vi "LVClass_SlopesPostProcessList ctor from copy.vi"(0 "SlopesPostProcessorList (const)":refnum<class "SlopesPostProcessorList.lvclass">, 5 "Dimensions_um":T1={"Size"={"X"=32, "Y"=32}, "Step"={"X"=1.0, "Y"=1.0}}, 7 "serial":string="7102", 9 "SlopesPostProcessorList to copy":refnum<class "SlopesPostProcessorList.lvclass">, 11 "error in (no error)":errorcluster) -> (4 "SlopesPostProcessorList (new)":refnum<class "SlopesPostProcessorList.lvclass">, 10 "SlopesPostProcessorList to copy (dup)":refnum<class "SlopesPostProcessorList.lvclass">, 15 "error out":errorcluster)   [LabVIEW 2020, in "SlopesPostProcessorList.lvclass"]
doc: "SlopesPostProcessorList constructor from copy.\n\n--------------------------------------------------------------------------------\n\n<B>NewSlopesPostProcessorListIn</B> : Constant Pointer to SlopesPostProcessorList object.\n<B>NewSlopesPostProcessorListOut</B> : Constant Pointer to SlopesPostProcessorList object.\n<B>SlopesPostProcessorListSrc </B> : SlopesPostProcessorList source object.\n<B>ErrorIn </B> : Error\n<B>ErrorOut </B> : Error\n\n--------------------------------------------------------------------------------"
uses:
  SlopesPostProcessorList.lvclass
  General dimensions definition.ctl
  Point2D.ctl
  Point2Df.ctl
  Handle creation.ctl
  SlopesPostProcessorList.lvclass/SlopesPostProcessorList.ctl
  HasoSlopes.lvclass
  Pupil.lvclass
  LVClass_SlopesPostProcessList Read SlopesPostProccessor.vi
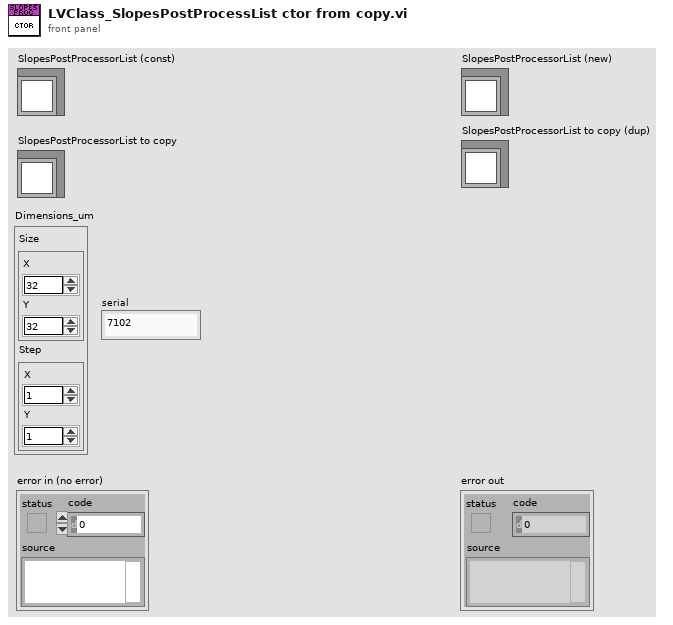
[diagram p1: front panel]
types:
  T1 = typedef "General dimensions definition.ctl" = cluster{"Size":T2, "Step":T3}
  T2 = typedef "Point2D.ctl" = cluster{"X":u32, "Y":u32}
  T3 = typedef "Point2Df.ctl" = cluster{"X":sgl, "Y":sgl}
  T4 = typedef "Handle creation.ctl" = enum16{"By ctor", "By write function"}
  T5 = typedef "ClassID.ctl" = i64
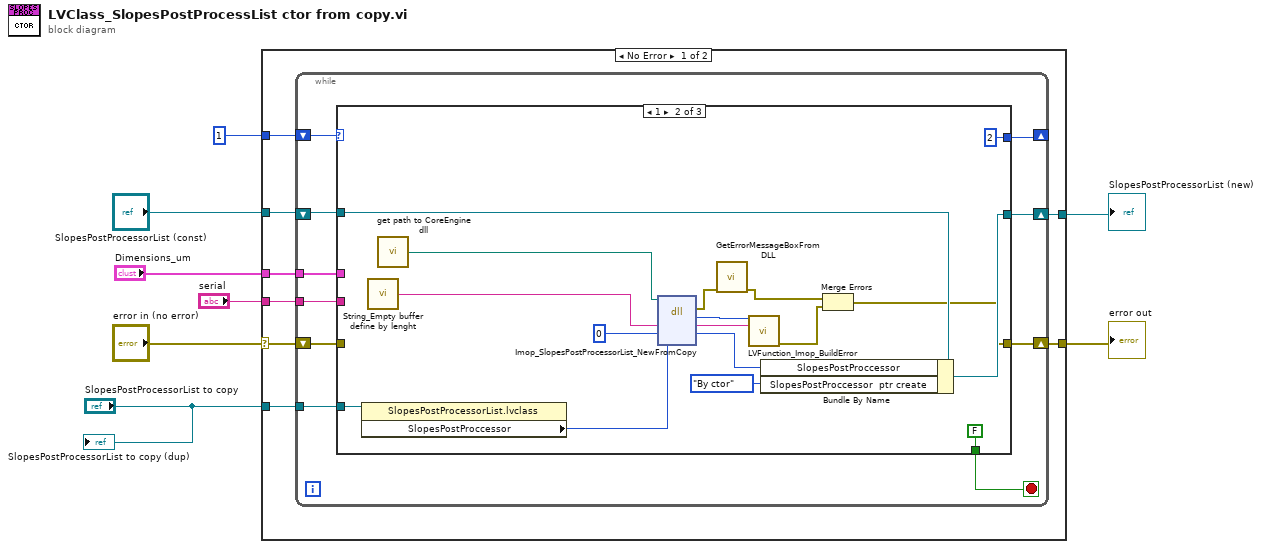
[diagram p0: block diagram]
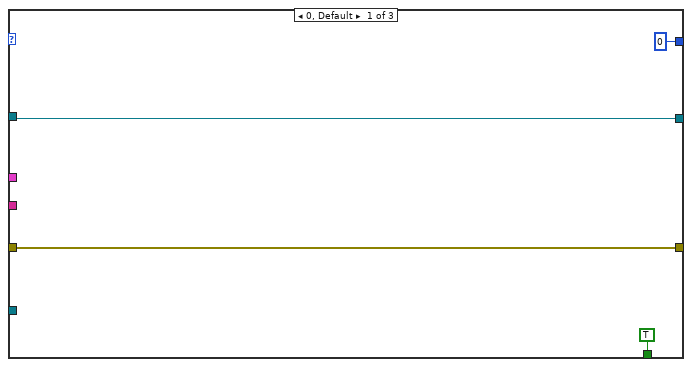
[diagram p2: hidden frame]
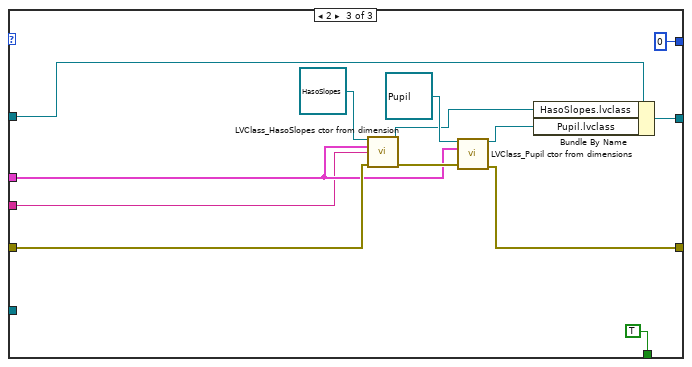
[diagram p3: hidden frame]
diagram:
  n1 = case shown="No Error" "error in (no error)" {
    selector: "error in (no error)" -> [w12 w61]
    tunnel: "SlopesPostProcessorList (const)" -> [w14 w62]
    tunnel: [w16 w62] -> w6
    tunnel: [w15 w61] -> w5
    tunnel: 1 -> [w13 _]
    tunnel: "Dimensions_um" -> [w11 _]
    tunnel: "serial" -> [w10 _]
    tunnel: "SlopesPostProcessorList to copy" -> [w9 _]
    frame No Error {
      n2 = while {
        shift-right: [w22] -> _
        shift-left: w13 -> [w23]
        shift-right: [w25] -> w15
        shift-left: w12 -> [w21]
        shift-right: [w26] -> w16
        shift-left: w14 -> [w24]
        tunnel: w11 -> [w19]
        tunnel: w10 -> [w18]
        tunnel: w9 -> [w17]
        stop <- w20 stop-if-true
        n3 = case shown="1" w23 {
          tunnel: [w28 w43 w52] -> w26
          tunnel: [w29 w33 w56] -> w25
          tunnel: w24 -> [w28 w42 w55]
          tunnel: [0 2 0] -> w22
          tunnel: w21 -> [w29 _ w59]
          tunnel: [TRUE FALSE TRUE] -> w20
          tunnel: w19 -> [_ _ w49]
          tunnel: w18 -> [_ _ w48]
          tunnel: w17 -> [_ w32 _]
          frame 0, Default {
          }
          frame 1 {
            n4 = property class="SlopesPostProcessorList.lvclass"(reference=w32) -> ("SlopesPostProccessor"=w31:T5)  [unwired: 1 in, 2 out]
            n5 = call "String_Empty buffer define by lenght.vi"() -> ("Empty buffer"=w47:string)  [unwired: 1 in]
            n6 = call "get path to CoreEngine dll.vi"() -> ("path to wavekit library"=w38:path)  [unwired: 14 in, 1 out]
            n7 = dll-call lib="D:/soft/HASO_v3/SVN_trunk/ImOpCoreEngine4_LV2011/DLLs/c_interface_vc100.dll" fn="Imop_SlopesPostProcessorList_NewFromCopy"(path in=w38, "message"=w47, "NewSlopesPostProcessor"=0 ("objet"), "SlopesPostProcessor"=w31) -> (error out=w41:errorcluster, "return type"=w44:i32, "message"=w45:string, "NewSlopesPostProcessor"=w46:i64)  [unwired: 3 in, 1 out]
            n8 = call "GetErrorMessageBoxFromDLL.vi"("error IN"=w41) -> ("error OUT"=w35:errorcluster)  [unwired: 10 in]
            n9 = call "LVFunction_Imop_BuildError.vi"("code"=w44, "String to Prepend to source (\"\")"=w45) -> ("error out"=w34:errorcluster)  [unwired: 13 in]
            n10 = Bundle By Name(cluster=w42, "SlopesPostProccessor"=w46, "SlopesPostProccessor  ptr create"=Handle_creation."By ctor" ("Slopes PP  ptr create")) -> (w43:refnum<class "SlopesPostProcessorList.lvclass">)
            n11 = Merge Errors(w35, w34) -> (w33:errorcluster)
          }
          frame 2 {
            n12 = call "LVClass_HasoSlopes ctor from dimension.vi"("HasoSlopes (const)"=refnum<class "HasoSlopes.lvclass"> refnum ("HasoSlopes in"), "Dimensions_um"=w49, "serial"=w48, "error in (no error)"=w59) -> ("HasoSlopes (new)"=w54:refnum<class "HasoSlopes.lvclass">, "error out"=w58:errorcluster)  [unwired: 10 in]
            n13 = call "LVClass_Pupil ctor from dimensions.vi"("Pupil (const)"=refnum<class "Pupil.lvclass"> refnum ("Pupil in"), "Dimensions_um"=w49, "error in (no error)"=w58) -> ("Pupil (new)"=w53:refnum<class "Pupil.lvclass">, "error out"=w56:errorcluster)  [unwired: 11 in]
            n14 = Bundle By Name(cluster=w55, "HasoSlopes.lvclass"=w54, "Pupil.lvclass"=w53) -> (w52:refnum<class "SlopesPostProcessorList.lvclass">)
          }
        }
      }
    }
    frame Error {
    }
  }
  "error out" <- w5
  "SlopesPostProcessorList (new)" <- w6
  "SlopesPostProcessorList to copy (dup)" <- "SlopesPostProcessorList to copy"
